vi "Cast 1D to 2D.vi"(1 "1D Monkeys":T1[](array[typedef])) -> (0 "2D Monkeys":T1[][](array[typedef]))   [LabVIEW 2020, in "Tamer.lvlib" / "Tamer.lvclass"]
uses:
  Tamer.lvclass
  Monkey Summary.ctl
  Run Utilities/TypeDefs/Monkey Status.ctl
  Link Chain GUI.ctl
  Run Utilities/Run Utilities.lvlib
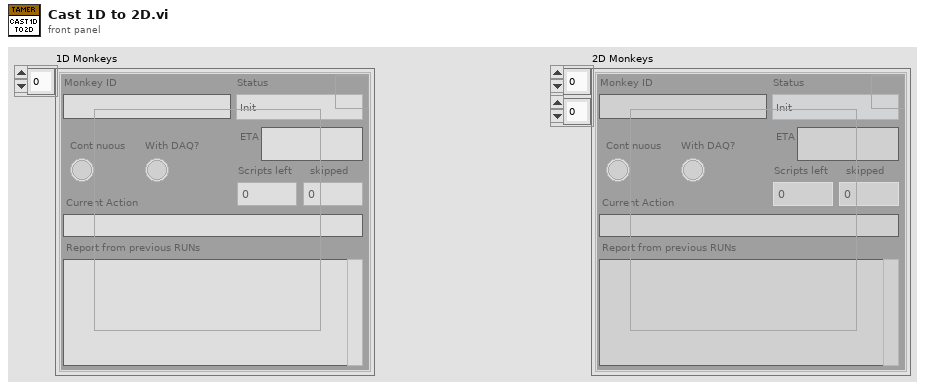
[diagram p1: front panel]
types:
  T1 = typedef "Tamer.lvlib/Tamer.lvclass/Monkey Summary.ctl" = cluster{"Color":u32, "Status":T2, "Continuous":bool, "Scripts left":u32, "Scripts skipped":u32, "ETA":string, "Current Action":string, "Report from previous RUNs":string, "Monkey ID":string, "With DAQ?":bool, "Linked?":T3, "Paused":bool}
  T2 = typedef "TALOS.lvlib/Run Utilities.lvlib/Monkey Status.ctl" = enum16{"Init", "Paused", "Ongoing", "Stopped", "Finished (no errors)", "Finished (with errors)"}
  T3 = typedef "Tamer.lvlib/Tamer.lvclass/Link Chain GUI.ctl" = bool
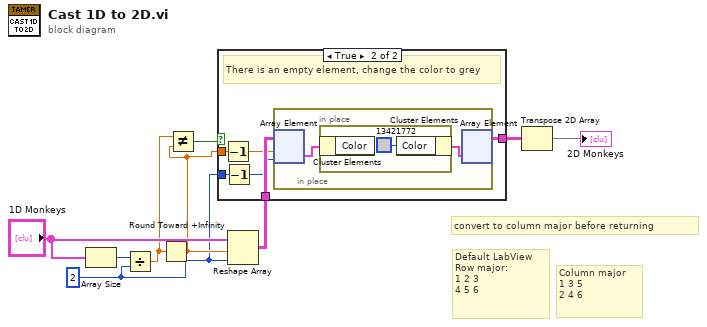
[diagram p0: block diagram]
diagram:
  w1 = 2 ("dimension size")
  # "Column major\n1 3 5\n2 4 6"
  # "Default LabView\nRow major:\n1 2 3\n4 5 6"
  # "convert to column major before returning"
  n1 = Array Size(array="1D Monkeys") -> (size(s)=w8:i32)
  n2 = Divide(x=w8, y=w1) -> (x/y=w5:dbl)
  n3 = Round Toward +Infinity(x=w5) -> (ceil(x): smallest int >= x=w2:dbl)
  n4 = Not Equal?(x=w5, y=w2) -> (x != y?=w6:bool)
  n5 = Reshape Array("1D Monkeys", w2, w1) -> (w3:T1[][])
  n6 = case shown="True" w6 {
    tunnel: w3 -> [w10 w16]
    tunnel: w1 -> [_ w15]
    tunnel: w2 -> [_ w12]
    tunnel: [w10 w11] -> w7
    frame False {
    }
    frame True {
      # "There is an empty element, change the color to grey"
      n7 = Decrement(x=w12) -> (x-1=w13:dbl)
      n8 = Decrement(x=w15) -> (x-1=w14:i32)
      n9 = in-place {
        n10 = in-place-array #1(w16, w13, w14) -> (w18:T1)
        n11 = in-place {
          n12 = in-place-cluster #2(w18) -> ()  [unwired: 1 out]
          n13 = in-place-cluster #2("Color"=u32 13421772) -> (w17:T1)
        }
        n14 = in-place-array #1(w17) -> (w11:T1[][])  [unwired: 2 out]
      }
    }
  }
  n15 = Transpose 2D Array(2D array=w7) -> (transposed array=→"2D Monkeys":T1[][])
